vi "Dumb Multimeter.vi"(1 "Action":T3=enum."Identify", 2 "Parameters":variant) -> (6 "Output":variant, 7 "Stop":bool)   [LabVIEW 2019]
uses:
  Sub Controls/Instrument Actions.ctl
  Sub Controls/Public.ctl
  Sub Controls/Instrument Match.ctl
  Sub Controls/User Event Command.ctl
  Sub Controls/Scan Output.ctl
panel:
  in  "Instruments":T1[](array[typedef])=[{"Model"=".*", "Manufacturer"=".*", "Term Character"="", "Wait Time (mS)"=0, "Wait for SRQ"=FALSE, "Type"="DumbMultimeter"}]
  in  "VISA resource name":refnum<visa-resource-name>
  in  "Address":u16(ring)
  out "Title":string="Dumb Multimeter"
  in  "Public":T2
  out "Measurement":dbl[](array[numeric]) format="%^_7e"
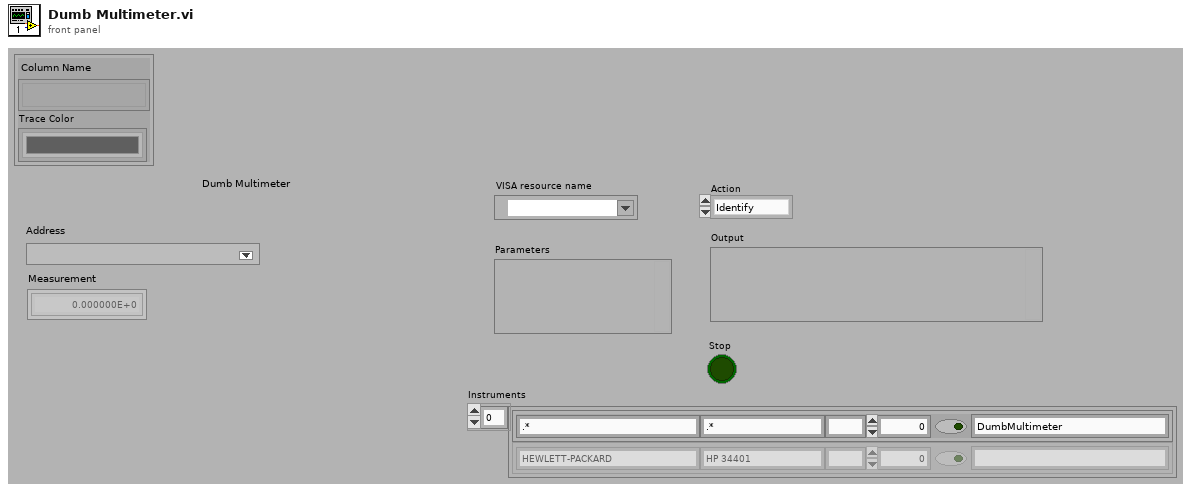
[diagram p1: front panel]
types:
  T1 = typedef "Instrument Match.ctl" = cluster{"Model":string, "Manufacturer":string, "Term Character":string, "Wait Time (mS)":u32, "Wait for SRQ":bool, "Type":string}
  T2 = typedef "Public.ctl" = cluster{"Column Name":string[], "Trace Color":u32[]}
  T3 = typedef "Instrument Actions.ctl" = enum16{"Scan", "Identify", "New", "Configure", "Initialize", "Test", "Read", "Close"}
  T4 = typedef "User Event Command.ctl" = enum32{"Stop Config"}
  T5 = typedef "Scan Output.ctl" = cluster{"Manufacturer":string, "Model":string, "Info":string, "Revision":string, "error out":errorcluster}
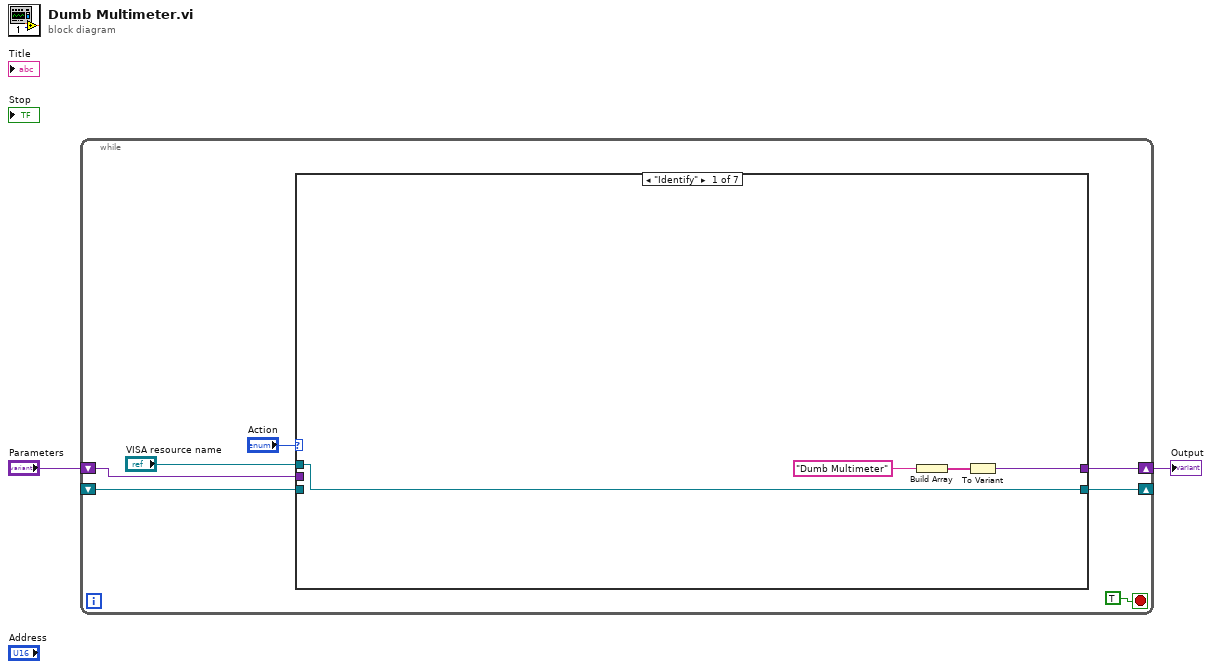
[diagram p0: block diagram]
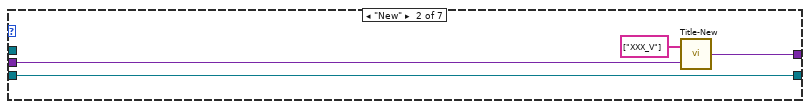
[diagram p2: hidden frame]
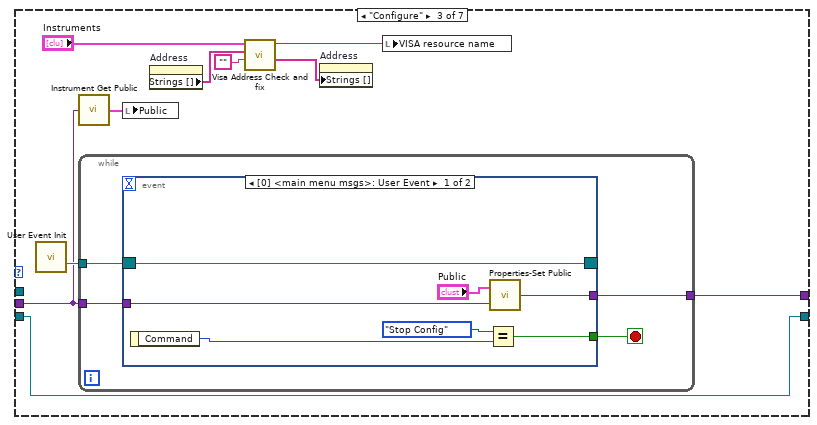
[diagram p3: hidden frame]
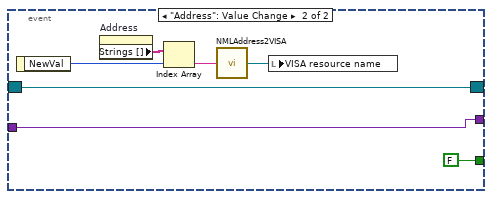
[diagram p4: hidden frame]
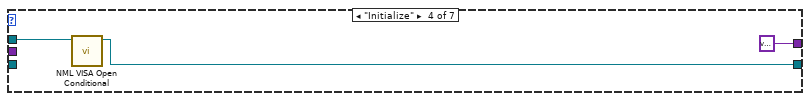
[diagram p5: hidden frame]
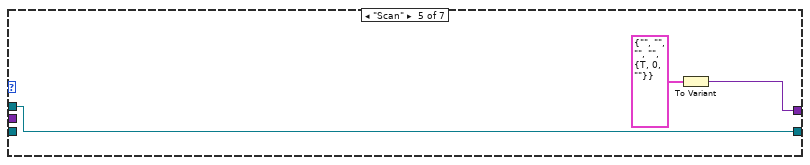
[diagram p6: hidden frame]
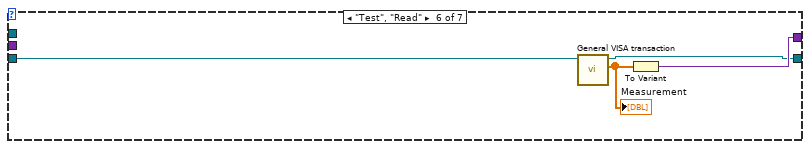
[diagram p7: hidden frame]
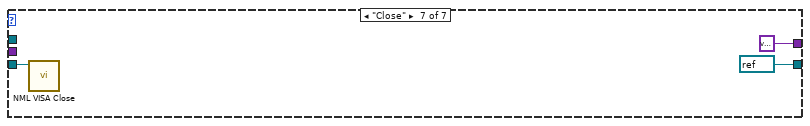
[diagram p8: hidden frame]
diagram:
  n1 = while {
    shift-right: [w8] -> w2
    shift-left: "Parameters" -> [w7]
    shift-right: [w3] -> _
    shift-left: _ -> [w5]
    stop <- TRUE stop-if-true
    n2 = case shown="\"Identify\"" "Action" {
      tunnel: [w12 w16 w27 variant ("Variant") w51 w55 variant ("Variant")] -> w8
      tunnel: w7 -> [_ w15 w24 _ _ _ _]
      tunnel: w5 -> [_ w14 w20 _ _ w54 w57]
      tunnel: "VISA resource name" -> [w10 _ _ w47 w49 _ _]
      tunnel: [w10 w14 w20 w46 w49 w53 refnum<visa-resource-name> refnum ("dup VISA session")] -> w3
      frame "Identify" {
        n3 = Build Array("Dumb Multimeter") -> (w11:string[])
        n4 = To Variant(anything=w11) -> (Variant=w12:variant)
      }
      frame "New" {
        n5 = call "Title-New.vi"("Parameters"=w15, "Array"=string[] ["XXX_V"]) -> ("Instrument Prop"=w16:variant)
      }
      frame "Configure" {
        n6 = call "User Event Init.vi"() -> ("Event Registration Refnum"=w25:refnum<event-registration>)  [unwired: 14 in, 1 out]
        n7 = call "Instrument Get Public.vi"("Variant"=w24) -> ("Public"=w26:T2)
        n8 = while {
          tunnel: w24 -> [w31]
          tunnel: [w30] -> w27
          tunnel: w25 -> [w28]
          stop <- w29 stop-if-true
          n9 = event shown="[0] <main menu msgs>: User Event" {
            selector: w28 -> [w32 w43]
            dyn-events: [w32 w43] -> _
            timeout: _ -> [_ _]
            tunnel: [w38 w44] -> w30
            tunnel: [w34 FALSE ("NewVal")] -> w29
            tunnel: w31 -> [w37 w44]
            event User Event {
              n10 = event-data() -> ("Command"=w36:T4)  [unwired: 1 in]
              n11 = Equal?(x=User_Event_Command."Stop Config", y=w36) -> (x = y?=w34:bool)
              n12 = call "Properties-Set Public.vi"("Variant"=w37, "New Public"="Public") -> ("Variant 2"=w38:variant)
            }
            event "Address": Value Change {
              n13 = event-data() -> ("NewVal"=w40:u16)  [unwired: 1 in]
              n14 = property on="Address" class="Ring (strict)"() -> ("Strings []"=w39:string[])  [unwired: 2 in, 2 out]
              n15 = Index Array(array=w39, index=w40) -> (element=w42:string)
              n16 = call "NMLAddress2VISA.vi"("NML Address"=w42) -> ("VISA resource name"=w41:refnum<visa-resource-name>)
              n17 = local write "VISA resource name"(w41) -> ()
            }
          }
        }
        n18 = local write "Public"(w26) -> ()
        n19 = property on="Address" class="Ring (strict)"() -> ("Strings []"=w23:string[])  [unwired: 2 in, 2 out]
        n20 = call "Visa Address Check and fix.vi"("Name"="", "NML Addresses"=w23, "Instruments"="Instruments") -> ("NML Addresses"=w21:string[], "VISA resource name"=w19:refnum<visa-resource-name>)  [unwired: 1 in, 4 out]
        n21 = property on="Address" class="Ring (strict)"("Strings []"=w21) -> ()  [unwired: 2 in, 2 out]
        n22 = local write "VISA resource name"(w19) -> ()
      }
      frame "Initialize" {
        n23 = call "NML VISA Open Conditional.vi"("VISA resource name"=w47) -> ("dup VISA Session"=w46:refnum<visa-resource-name>)  [unwired: 8 in, 2 out]
      }
      frame "Scan" {
        n24 = To Variant(anything=T5 {"Manufacturer"="", "Model"="", "Info"="", "Revision"="", "error out"={"status"=TRUE, "code"=0, "source"=""}} ("Scan Output")) -> (Variant=w51:variant)
      }
      frame "Test", "Read" {
        n25 = call "General VISA transaction.vi"("VISA Session"=w54) -> ("Measurement"=w52:dbl[], "dup VISA Session"=w53:refnum<visa-resource-name>)  [unwired: 5 in, 4 out]
        "Measurement" <- w52
        n26 = To Variant(anything=w52) -> (Variant=w55:variant)
      }
      frame "Close" {
        n27 = call "NML VISA Close.vi"("VISA resource name"=w57) -> ()  [unwired: 10 in, 1 out]
      }
    }
  }
  "Output" <- w2
